vi "test Run Rx Asynchronously.vi"(8 "error in (no error)":errorcluster) -> (0 "error out":errorcluster)   [LabVIEW 2020, in "Create Execution Unit.lvclass"]
uses:
  Create Execution Unit.lvclass
  <vilib>/addons/_JKI Toolkits/VI Tester/TestCase.llb/TestCase.lvclass
  Scripting/AIM MIL-STD-1553 Scripting.lvlib
  Engine/Implementation/Execution Unit Factory/Execution Unit Factory.lvclass
  C:/Program Files (x86)/National Instruments/LabVIEW 2020/vi.lib/addons/_JKI Toolkits/VI Tester/TestCase.llb/TestCase.lvclass
panel:
  in  "TestCase in":refnum<class "Create Execution Unit.lvclass">
  out "TestCase out":refnum<class "Create Execution Unit.lvclass">
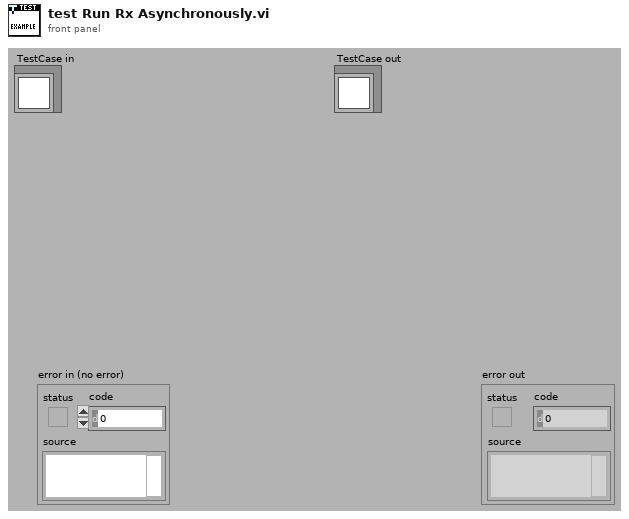
[diagram p1: front panel]
types:
  T1 = typedef "Custom Device API.lvlib/Custom Device Item Ref.ctl" = u64
  T2 = typedef "AIM MIL-STD-1553 Engine.lvlib/Interfaces.lvlib/Execution Unit Information.ctl" = cluster{"Execution Unit":refnum<class "Execution Unit.lvclass">, "Incoming Channels":T1[], "Outgoing Channels":T1[], "ReadWrite Channels":T1[]}
  T3 = cluster{"grouped asynchronous execution units":T2[]}[]
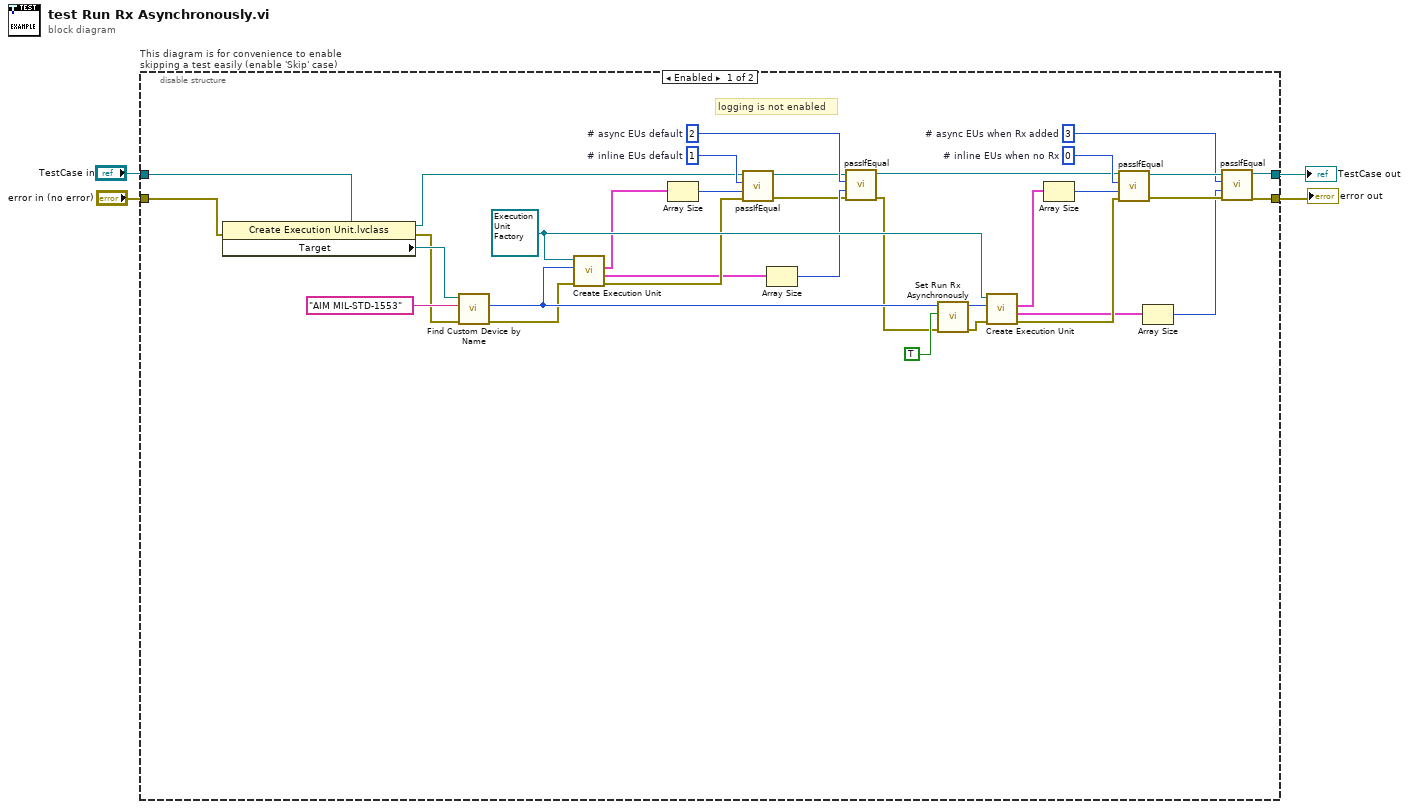
[diagram p0: block diagram]
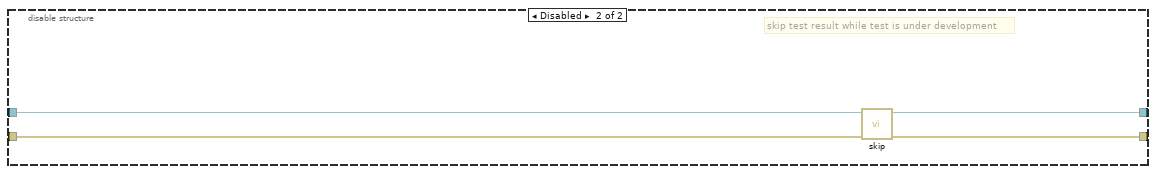
[diagram p2: hidden frame]
diagram:
  n1 = disable-structure "This diagram is for convenience to enable skipping a test easily (enable 'Skip' case)" shown="Enabled" {
    disable-tunnel: "TestCase in" -> [w37 w42]
    disable-tunnel: [w20 w40] -> w1
    disable-tunnel: [w21 w41] -> w3
    disable-tunnel: "error in (no error)" -> [w36 w39]
    frame Enabled {
      w16 = 2  # # async EUs default
      w11 = 1  # # inline EUs default
      w19 = refnum<class "Execution Unit Factory.lvclass"> refnum ("Communication Bus Template Interfaces:Implementation.lvlib:Execution Unit Factory.lvclass")
      w23 = 3  # # async EUs when Rx added
      w28 = 0  # # inline EUs when no Rx
      # "logging is not enabled"
      n2 = property class="Create Execution Unit.lvclass"(reference=w37, error in=w36) -> (reference out=w6:refnum<class "Create Execution Unit.lvclass">, error out=w31:errorcluster, "Target"=w35:refnum<k24>)
      n3 = call "Find Custom Device by Name.vi"("error in"=w31, "custom device name"="AIM MIL-STD-1553", "target"=w35) -> ("error out"=w17:errorcluster, "custom device"=w18:T1)  [unwired: 5 in, 2 out]
      n4 = call-dynamic "Create Execution Unit.vi"("error in"=w17, "custom device ref"=w18, "execution unit factory"=w19) -> ("error out"=w10:errorcluster, "asynchronous execution units"=w9:T3, "inline execution units"=w8:T2[])  [unwired: 5 in, 1 out]
      n5 = Array Size(array=w8) -> (size(s)=w12:i32)
      n6 = call-dynamic "passIfEqual.vi"("error in (no error)"=w10, "y"=w12, "x"=w11, "TestCase in"=w6) -> ("error out"=w14:errorcluster, "TestCase out"=w13:refnum<class "Create Execution Unit.lvclass">)  [unwired: 6 in]
      n7 = Array Size(array=w9) -> (size(s)=w15:i32)
      n8 = call-dynamic "passIfEqual.vi"("error in (no error)"=w14, "y"=w15, "x"=w16, "TestCase in"=w13) -> ("error out"=w7:errorcluster, "TestCase out"=w5:refnum<class "Create Execution Unit.lvclass">)  [unwired: 6 in]
      n9 = call "Set Run Rx Asynchronously.vi"("error in"=w7, "run rx asynchronously"=TRUE, "custom device"=w18) -> ("error out"=w32:errorcluster, "custom device out"=w33:T1)  [unwired: 7 in]
      n10 = call-dynamic "Create Execution Unit.vi"("error in"=w32, "custom device ref"=w33, "execution unit factory"=w19) -> ("error out"=w30:errorcluster, "asynchronous execution units"=w22:T3, "inline execution units"=w29:T2[])  [unwired: 5 in, 1 out]
      n11 = Array Size(array=w29) -> (size(s)=w27:i32)
      n12 = call-dynamic "passIfEqual.vi"("error in (no error)"=w30, "y"=w27, "x"=w28, "TestCase in"=w5) -> ("error out"=w25:errorcluster, "TestCase out"=w26:refnum<class "Create Execution Unit.lvclass">)  [unwired: 6 in]
      n13 = Array Size(array=w22) -> (size(s)=w24:i32)
      n14 = call-dynamic "passIfEqual.vi"("error in (no error)"=w25, "y"=w24, "x"=w23, "TestCase in"=w26) -> ("error out"=w21:errorcluster, "TestCase out"=w20:refnum<class "Create Execution Unit.lvclass">)  [unwired: 6 in]
    }
    frame Disabled {
      # "skip test result while test is under development"
      n15 = call <vilib>:"skip.vi"("error in (no error)"=w39, "TestCase in"=w42) -> ("error out"=w41:errorcluster, "TestCase out"=w40:refnum<class "Create Execution Unit.lvclass">)  [unwired: 8 in]
    }
  }
  "error out" <- w3
  "TestCase out" <- w1
